vi "ROIsToSelCells.vi"(10 "Scan Settings":T2, 11 "ROI":T1(array[cluster])) -> (2 "Number of points":i32, 3 "Points_um":dbl[][](array[numeric]))   [LabVIEW 2014]
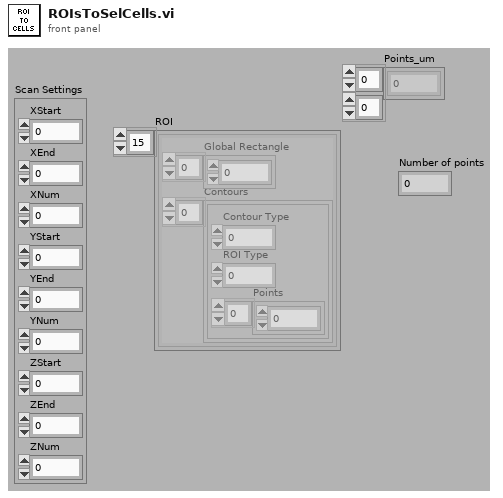
[diagram p1: front panel]
types:
  T1 = cluster{"Global Rectangle":i32[], "Contours":cluster{"Contour Type":u32, "ROI Type":u32, "Points":i32[]}[]}[]
  T2 = cluster{"XStart":dbl, "XEnd":dbl, "XNum":dbl, "YStart":dbl, "YEnd":dbl, "YNum":dbl, "ZStart":dbl, "ZEnd":dbl, "ZNum":dbl}
  T3 = cluster{"Contour Type":u32, "ROI Type":u32, "Points":i32[]}[]
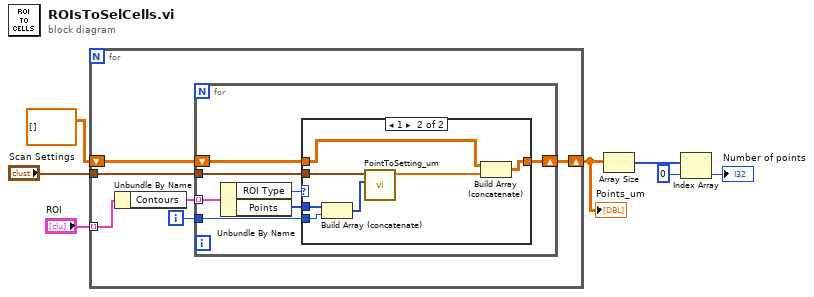
[diagram p0: block diagram]
diagram:
  n1 = for {
    tunnel: "ROI" -> [w13] mode=indexing
    shift-right: [w10] -> w2
    shift-left: dbl[][] [] -> [w11]
    tunnel: "Scan Settings" -> [w9]
    i -> [w8]
    n2 = Unbundle By Name(w13) -> ("Contours"=w12:T3)
    n3 = for {
      tunnel: w12 -> [w20] mode=indexing
      shift-right: [w16] -> w10
      shift-left: w11 -> [w17]
      tunnel: w9 -> [w15]
      tunnel: w8 -> [w14]
      n4 = Unbundle By Name(w20) -> ("ROI Type"=w19:u32, "Points"=w18:i32[])
      n5 = case shown="1" w19 {
        tunnel: w18 -> [_ w26]
        tunnel: w17 -> [w21 w28]
        tunnel: [w21 w27] -> w16
        tunnel: w15 -> [_ w24]
        tunnel: w14 -> [_ w25]
        frame 0, Default {
        }
        frame 1 {
          n6 = Build Array (concatenate)(w26, w25) -> (w23:i32[])
          n7 = call "PointToSetting_um.vi"("Clicked"=w23, "Scan Settings"=w24) -> ("Setting"=w22:dbl[])  [unwired: 9 in]
          n8 = Build Array (concatenate)(w28, w22) -> (w27:dbl[][])
        }
      }
    }
  }
  "Points_um" <- w2
  n9 = Array Size(array=w2) -> (size(s)=w5:i32[])
  n10 = Index Array(array=w5, index=0) -> (element=→"Number of points":i32)
